vi "Draw Plot Image.vi"(4 "pen":T1, 6 "Plot Color":u32(colorbox), 7 "Plot Vertex":cluster{"X":i16, "Y":i16}[][](array[cluster]), 11 "Picture In":picture) -> (3 "Picture Out":picture)   [LabVIEW 2020, in "2D Plot.lvclass"]
uses:
  <vilib>/Math Plots/2D Math Plots/2D Plot/2D Plot/2D Plot.lvclass
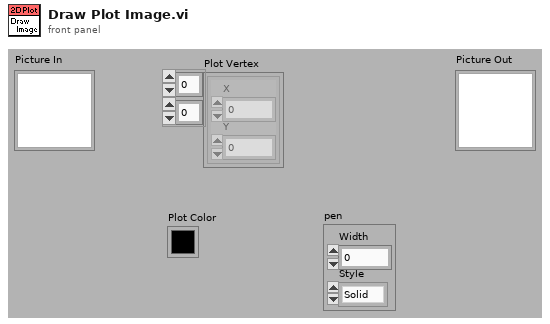
[diagram p1: front panel]
types:
  T1 = cluster{"Width":u16, "Style":enum32{"Solid", "Dash", "Dot", "DashDot", "DashDotDot"}}
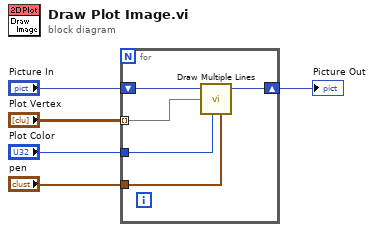
[diagram p0: block diagram]
diagram:
  n1 = for {
    shift-right: [w10] -> w4
    shift-left: "Picture In" -> [w7]
    tunnel: "Plot Vertex" -> [w9] mode=indexing
    tunnel: "Plot Color" -> [w8]
    tunnel: "pen" -> [w6]
    n2 = call <vilib>:"Draw Multiple Lines.vi"("picture"=w7, "line endpoints"=w9, "color(black)"=w8, "pen"=w6) -> ("new picture"=w10:picture)  [unwired: 1 in, 4 out]
  }
  "Picture Out" <- w4
